vi "DLTS - set bias (SubVI).vi"(8 "error in (no error)":errorcluster, 9 "AUX offset":dbl, 10 "AUX scale":dbl, 11 "ziHandle":T1 {"Handle" format="0x%08x"; "Conn" format="0x%08x"}) -> (0 "error out":errorcluster, 3 "Handle Out":T1 {"Handle" format="0x%08x"; "Conn" format="0x%08x"})   [LabVIEW 2019]
doc: "Sets biasing voltage for a DLTS measurement"
uses:
  <instrlib>/Zurich Instruments LabOne/Public/ziTypeHandle.ctl
  <instrlib>/Zurich Instruments LabOne/Public/Configure/ziSetValueDoubleArray.vi
  <instrlib>/Zurich Instruments LabOne/Zurich Instruments LabOne.lvlib
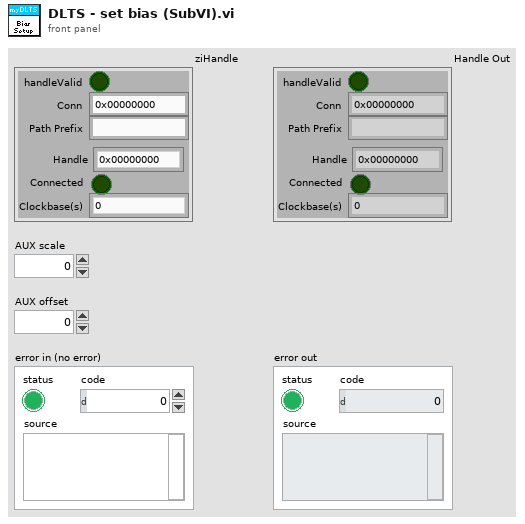
[diagram p1: front panel]
types:
  T1 = typedef "Zurich Instruments LabOne.lvlib/ziTypeHandle.ctl" = cluster{"handleValid":bool, "Conn":u64, "Path Prefix":string, "Handle":u64, "Connected":bool, "Clockbase(s)":dbl}
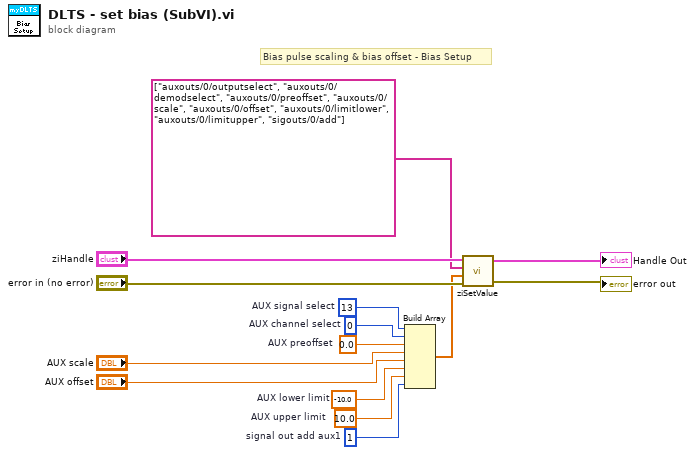
[diagram p0: block diagram]
diagram:
  w1 = 1  # signal out add aux1
  w6 = 10.0  # AUX upper limit
  w5 = -10.0  # AUX lower limit
  w4 = 0.0  # AUX preoffset
  w3 = 0  # AUX channel select
  w2 = 13  # AUX signal select
  # "Bias pulse scaling & bias offset - Bias Setup"
  n1 = Build Array(w2, w3, w4, "AUX scale", "AUX offset", w5, w6, w1) -> (w8:dbl[])
  n2 = call-poly <instrlib>:"ziSetValue.vi"("Error In"="error in (no error)", "Values"=w8, "Paths"=string[] ["auxouts/0/outputselect", "auxouts/0/demodselect", "auxouts/0/preoffset", "auxouts/0/scale", "auxouts/0/offset", "auxouts/0/limitlower", "auxouts/0/limitupper", "sigouts/0/add"], "Handle In"="ziHandle") -> ("Error Out"=→"error out":errorcluster, "Handle Out"=→"Handle Out":T1)  [unwired: 1 in]
